vi "kvCanReadSpecificSkip.vi"(6 "error in (no error)":errorcluster, 7 "Message Id":i32, 8 "Channel Handle (input only)":i32) -> (0 "Message Data":u8[](array[numeric]), 1 "error out":errorcluster, 2 "Message Timestamp":u32, 3 "Message Flags":u32, 5 "Channel Handle (output only)":i32)   [LabVIEW 2022 SP3]
doc: "Reads a message with a specified identifier from the receive buffer. Any preceeding message not matching the specified identifier will be removed in the receive buffer. If no message with the specified identifier is available, the function returns immediately with an error code."
uses:
  canlib32.dll
panel:
  # "8"
  # "16"
  # "24"
  # "32"
  # "40"
  # "48"
  # "56"
  # "64"
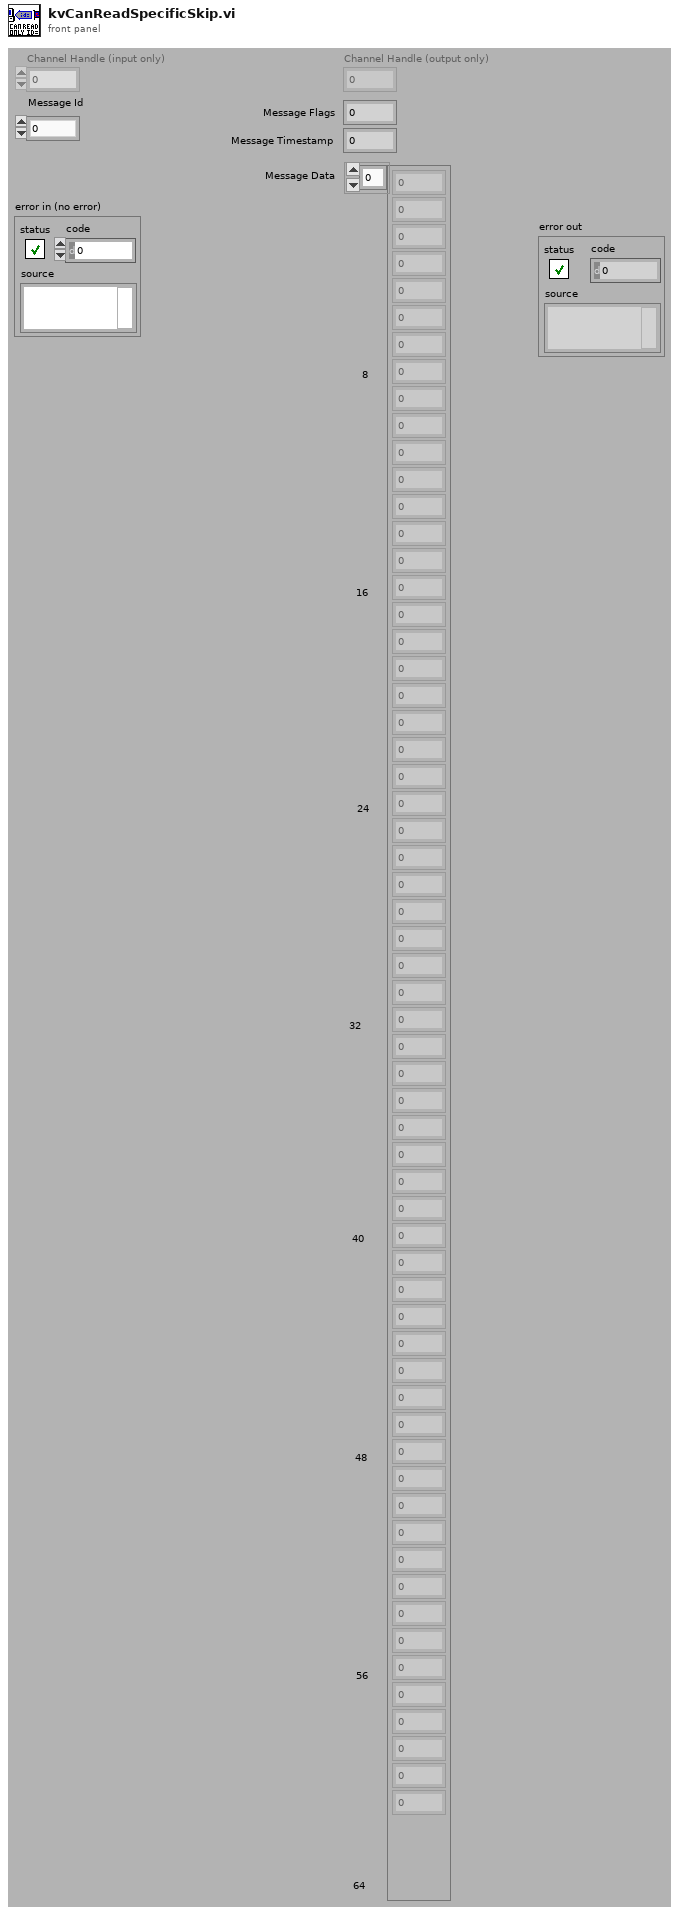
[diagram p1: front panel]
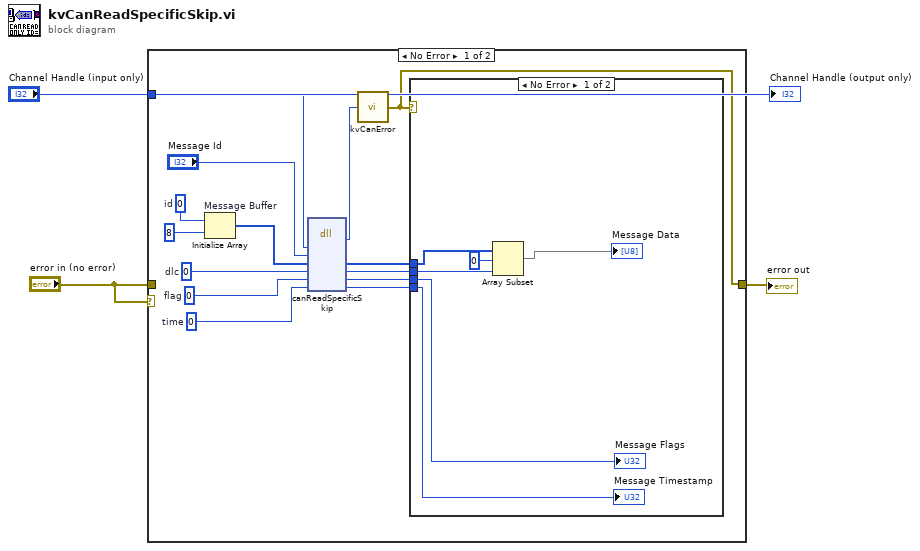
[diagram p0: block diagram]
diagram:
  n1 = case shown="No Error" "error in (no error)" {
    tunnel: [w5 w24] -> w2
    tunnel: "error in (no error)" -> [_ w24]
    tunnel: "Channel Handle (input only)" -> [w17 _]
    frame No Error {
      w13 = 0  # time
      w12 = 0  # flag
      w11 = 0  # dlc
      w16 = 0  # id
      n2 = Initialize Array "Message Buffer"(w16, 8) -> (w14:i32[])
      n3 = dll-call lib="canlib32.dll" fn="canReadSpecificSkip"("handle"=w17, "id"="Message Id", "msg"=w14, "dlc"=w11, "flag"=w12, "time"=w13) -> (w10:i32, "msg"=w6:u8[], "dlc"=w7:u32, "flag"=w8:u32, "time"=w9:u32)  [unwired: 5 in, 2 out]
      n4 = call "kvCanError.vi"("error code"=w10) -> ("error out"=w5:errorcluster)
      n5 = case shown="No Error" w5 {
        tunnel: w9 -> [w23 _]
        tunnel: w8 -> [w22 _]
        tunnel: w7 -> [w18 _]
        tunnel: w6 -> [w21 _]
        frame No Error {
          n6 = Array Subset(array=w21, index=u32 0, length=w18) -> (→"Message Data":u8[])
          "Message Timestamp" <- w23
          "Message Flags" <- w22
        }
        frame Error {
        }
      }
    }
    frame Error {
    }
  }
  "error out" <- w2
  "Channel Handle (output only)" <- "Channel Handle (input only)"
